vi "String Constant - One Line State String Wired to Add States.vi"   [LabVIEW 2013]
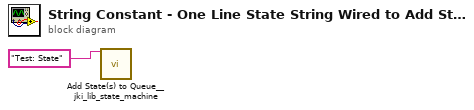
[diagram p0: block diagram]
diagram:
  n1 = call <vilib>:"Add State(s) to Queue__jki_lib_state_machine.vi"("State(s) in Front (\"\")"="Test: State") -> ()  [unwired: 14 in, 1 out]
